vi "Stop Core.vi"(10 "final error code":i32, 11 "TCPIP Reader in":refnum<class "TCPIP Reader.lvclass">) -> (3 "TCPIP Reader out":refnum<class "TCPIP Reader.lvclass">)   [LabVIEW 2015, in "TCPIP Reader Actor.lvlib" / "TCPIP Reader.lvclass"]
doc: "(<B>Filename</B>: Actor Framework.lvlib:Actor.lvclass:Stop Core.vi)\n\nDefines what the actor does before it stops. Use the <B>final error code</B> input to determine whether the actor shut down in response to an error.\n\nBy default, this method does nothing. A descendant class may override it to define behavior, such as shutting down any processes the actor initiated in its override of the Actor Core method."
uses:
  TCPIP Reader.lvclass
  TCPIP Reader.lvclass/TCPIP Reader.ctl
  <vilib>/ActorFramework/Actor/Actor.lvclass
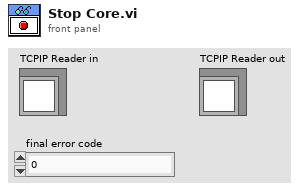
[diagram p1: front panel]
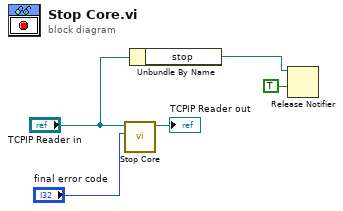
[diagram p0: block diagram]
diagram:
  n1 = call-parent "Stop Core.vi"("final error code"="final error code", "Actor in"="TCPIP Reader in") -> ("Actor out"=→"TCPIP Reader out":refnum<class "TCPIP Reader.lvclass">)  [unwired: 9 in]
  n2 = Unbundle By Name("TCPIP Reader in") -> ("stop"=w2:refnum<notifier>)
  n3 = Release Notifier(notifier=w2, force destroy? (F)=TRUE) -> ()  [unwired: 1 in, 3 out]
